vi "Create Collection.vi"(10 "Cache":refnum<class "ConfigManager.Cache.lvclass">, 11 "List":refnum<class "ConfigManager.lvclass">[](array[class])) -> (3 "SMOConfigManagerCollection out":refnum<class "ConfigManagerCollection.lvclass">)   [LabVIEW 2013, in "SMOConfig.lvlib" / "ConfigManagerCollection.lvclass"]
uses:
  ConfigManagerCollection.lvclass
  Manager/ConfigManager.lvclass
  Cache/ConfigManager.Cache.lvclass
  ConfigManagerCollection.lvclass/ConfigManagerCollection.ctl
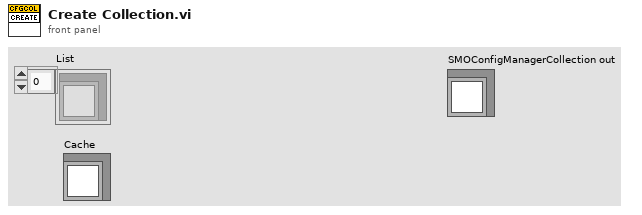
[diagram p1: front panel]
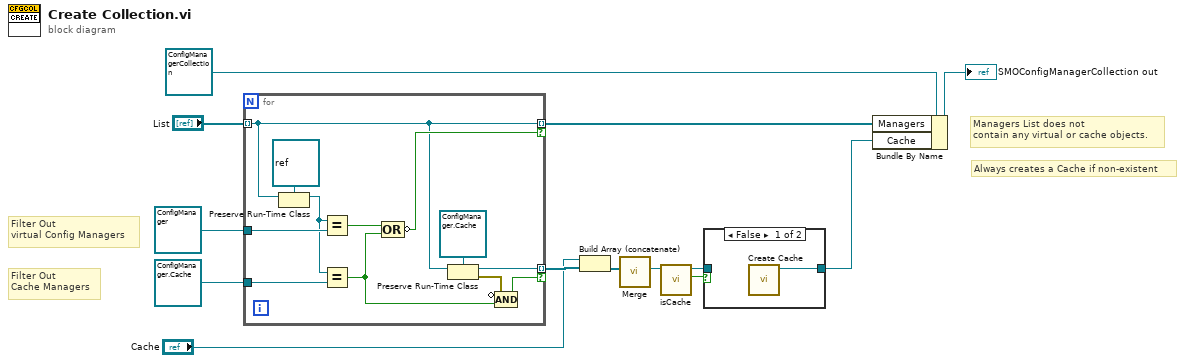
[diagram p0: block diagram]
diagram:
  # "Always creates a Cache if non-existent"
  # "Managers List does not\ncontain any virtual or cache objects."
  # "Filter Out\nCache Managers"
  # "Filter Out\nvirtual Config Managers"
  n1 = for {
    tunnel: "List" -> [w20] mode=indexing
    tunnel: refnum<class "ConfigManager.lvclass"> refnum ("SMOConfigManager.lvclass") -> [w25]
    tunnel: [w20] -> w8 mode=indexing if=w21
    tunnel: refnum<class "ConfigManager.Cache.lvclass"> refnum ("SMOConfig.lvlib:ConfigManager.Cache.lvclass") -> [w15]
    tunnel: [w19] -> w7 mode=indexing if=w16
    n2 = Preserve Run-Time Class(object in=w20, 2:refnum<class> refnum ("LabVIEW Object")) -> (object out=w23:refnum<class>)  [unwired: 1 in, 1 out]
    n3 = Equal?(x=w23, y=w25) -> (x = y?=w22:bool)
    n4 = Equal?(x=w23, y=w15) -> (x = y?=w17:bool)
    n5 = Compound Arithmetic op=OR(w22, w17) -> (invert w21:bool)
    n6 = Preserve Run-Time Class(object in=w20, 2:refnum<class "ConfigManager.Cache.lvclass"> refnum ("SMOConfig.lvlib:ConfigManager.Cache.lvclass")) -> (object out=w19:refnum<class "ConfigManager.Cache.lvclass">, error out=w18:errorcluster)  [unwired: 1 in]
    n7 = Compound Arithmetic op=AND(invert w18, w17) -> (w16:bool)
  }
  n8 = Build Array (concatenate)("Cache", w7) -> (w2:refnum<class "ConfigManager.Cache.lvclass">[])
  n9 = call "Merge.vi"("Cache Managers"=w2) -> ("Merged Cache"=w5:refnum<class "ConfigManager.Cache.lvclass">)  [unwired: 10 in]
  n10 = call "isCache.vi"("ConfigManager.Cache in"=w5) -> ("isCache?"=w4:bool, "ConfigManager.Cache out"=w3:refnum<class "ConfigManager.Cache.lvclass">)  [unwired: 9 in]
  n11 = case shown="False" w4 {
    tunnel: [w26 w27] -> w6
    tunnel: w3 -> [_ w27]
    frame False {
      n12 = call "Create Cache.vi"() -> ("ConfigManager.Cache"=w26:refnum<class "ConfigManager.Cache.lvclass">)  [unwired: 11 in]
    }
    frame True {
    }
  }
  n13 = Bundle By Name(cluster=refnum<class "ConfigManagerCollection.lvclass"> refnum ("SMOConfigManagerCollection.lvclass"), "Managers"=w8, "Cache"=w6) -> (→"SMOConfigManagerCollection out":refnum<class "ConfigManagerCollection.lvclass">)
